vi "ReadCamera.vi"(7 "Color":u16(ring) items=["Blue", "Green", "Red", "Orange", "Yellow"], 8 "error in":errorcluster) -> (0 "error out":errorcluster, 2 "Camera Data":dbl[][](array[numeric]) format="%.2f")   [LabVIEW 2018]
uses:
  <vilib>/vision/NI_Vision_Development_Module.lvlib
panel:
  out "Image":T1(plugin-control)
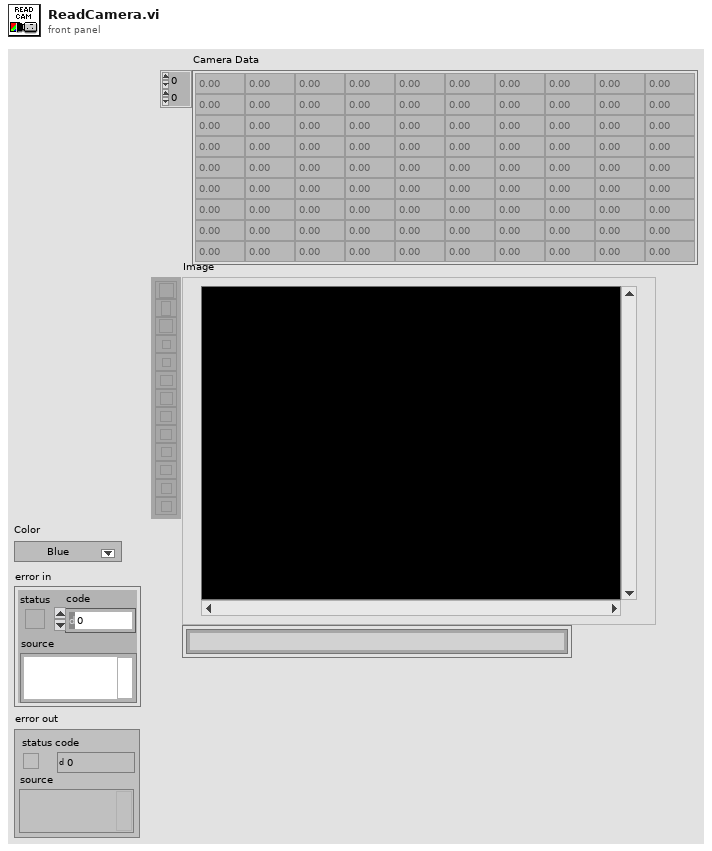
[diagram p1: front panel]
types:
  T1 = typedef "IMAQ Image.ctl" = refnum<image>
  T2 = typedef "Particle Parameters" = i32
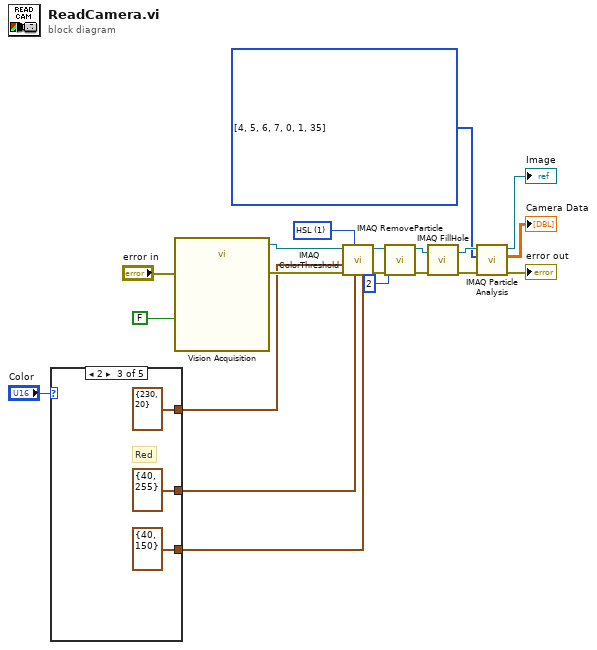
[diagram p0: block diagram]
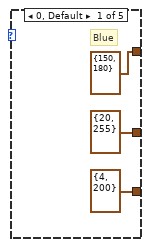
[diagram p2: hidden frame]
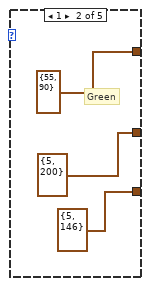
[diagram p3: hidden frame]
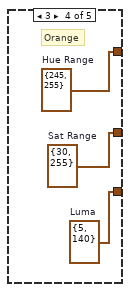
[diagram p4: hidden frame]
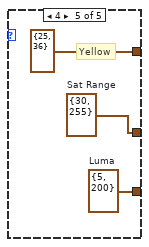
[diagram p5: hidden frame]
diagram:
  w7 = T2[] [4, 5, 6, 7, 0, 1, 35] items=["Center of Mass X", "Center of Mass Y", "First Pixel X", "First Pixel Y", "Bounding Rect Left", "Bounding Rect Top", "Bounding Rect Right", "Bounding Rect Bottom", "Max Feret Diameter Start X", "Max Feret Diameter Start Y", "Max Feret Diameter End X", "Max Feret Diameter End Y", "Max Horiz. Segment Length Left", "Max Horiz. Segment Length Right", "Max Horiz. Segment Length Row", "-", "Bounding Rect Width", "Bounding Rect Height", "Bounding Rect Diagonal", "Perimeter", "Convex Hull Perimeter", "Holes' Perimeter", "Max Feret Diameter", "Equivalent Ellipse Major Axis", "Equivalent Ellipse Minor Axis", "Equivalent Ellipse Minor Axis (Feret)", "Equivalent Rect Long Side", "Equivalent Rect Short Side", "Equivalent Rect Diagonal", "Equivalent Rect Short Side (Feret)", "Average Horiz. Segment Length", "Average Vert. Segment Length", "Hydraulic Radius", "Waddel Disk Diameter", "-", "Area", "Holes' Area", "Particle & Holes' Area", "Convex Hull Area", "Image Area", "-", "Number of Holes", "Number of Horiz. Segments", "Number of Vert. Segments", "-", "Orientation", "Max Feret Diameter Orientation", "-", "% Area/Image Area", "% Area/(Particle & Holes' Area)", "Ratio of Equivalent Ellipse Axes", "Ratio of Equivalent Rect Sides", "-", "Elongation Factor", "Compactness Factor", "Heywood Circularity Factor", "Type Factor", "-", "Sum X", "Sum Y", "Sum XX", "Sum XY", "Sum YY", "Sum XXX", "Sum XXY", "Sum XYY", "Sum YYY", "-", "Moment of Inertia XX", "Moment of Inertia XY", "Moment of Inertia YY", "Moment of Inertia XXX", "Moment of Inertia XXY", "Moment of Inertia XYY", "Moment of Inertia YYY", "Norm. Moment of Inertia XX", "Norm. Moment of Inertia XY", "Norm. Moment of Inertia YY", "Norm. Moment of Inertia XXX", "Norm. Moment of Inertia XXY", "Norm. Moment of Inertia XYY", "Norm. Moment of Inertia YYY", "Hu Moment 1", "Hu Moment 2", "Hu Moment 3", "Hu Moment 4", "Hu Moment 5", "Hu Moment 6", "Hu Moment 7"] ("Pixel Measurements")
  w17 = u16 1 items=["RGB", "HSL", "HSV", "HSI"] ("Color Mode")
  n1 = case shown="2" "Color" {
    tunnel: [cluster{"Lower value":i32, "Upper value":i32} {"Lower value"=150, "Upper value"=180} ("Hue Range") cluster{"Lower value":i32, "Upper value":i32} {"Lower value"=55, "Upper value"=90} ("Hue Range") cluster{"Lower value":i32, "Upper value":i32} {"Lower value"=230, "Upper value"=20} ("Hue Range") w32 cluster{"Lower value":i32, "Upper value":i32} {"Lower value"=25, "Upper value"=36} ("Hue Range")] -> w16
    tunnel: [cluster{"Lower value":i32, "Upper value":i32} {"Lower value"=20, "Upper value"=255} ("Sat Range") cluster{"Lower value":i32, "Upper value":i32} {"Lower value"=5, "Upper value"=200} ("Sat Range") cluster{"Lower value":i32, "Upper value":i32} {"Lower value"=40, "Upper value"=255} ("Sat Range") w31 w34] -> w15
    tunnel: [cluster{"Lower value":i32, "Upper value":i32} {"Lower value"=4, "Upper value"=200} ("Luma") cluster{"Lower value":i32, "Upper value":i32} {"Lower value"=5, "Upper value"=146} ("Luma") cluster{"Lower value":i32, "Upper value":i32} {"Lower value"=40, "Upper value"=150} ("Luma") w30 w33] -> w14
    frame 0, Default {
      # "Blue"
    }
    frame 1 {
      # "Green"
    }
    frame 2 {
      # "Red"
    }
    frame 3 {
      w30 = cluster{"Lower value":i32, "Upper value":i32} {"Lower value"=5, "Upper value"=140}  # Luma
      w31 = cluster{"Lower value":i32, "Upper value":i32} {"Lower value"=30, "Upper value"=255}  # Sat Range
      w32 = cluster{"Lower value":i32, "Upper value":i32} {"Lower value"=245, "Upper value"=255}  # Hue Range
      # "Orange"
    }
    frame 4 {
      w33 = cluster{"Lower value":i32, "Upper value":i32} {"Lower value"=5, "Upper value"=200}  # Luma
      w34 = cluster{"Lower value":i32, "Upper value":i32} {"Lower value"=30, "Upper value"=255}  # Sat Range
      # "Yellow"
    }
  }
  n2 = call "Vision Acquisition"("Stop (F)"=FALSE, "error in"="error in") -> ("Image Out"=w3:T1, "error out"=w18:errorcluster)  [unwired: 23 in, 1 out]
  n3 = call "IMAQ ColorThreshold"("Blue or Luma or Val or Inten Range"=w14, "Green or Sat Range"=w15, "Color Mode"=w17, "error in (no error)"=w18, "Red or Hue Range"=w16, "Image Src"=w3) -> ("error out"=w13:errorcluster, "Image Dst Out"=w12:T1)  [unwired: 4 in]
  n4 = call "IMAQ RemoveParticle"("error in (no error)"=w13, "Number of Erosion"=2, "Image Src"=w12) -> ("error out"=w11:errorcluster, "Image Dst Out"=w10:T1)  [unwired: 7 in]
  n5 = call "IMAQ FillHole"("error in (no error)"=w11, "Image Src"=w10) -> ("error out"=w9:errorcluster, "Image Dst Out"=w8:T1)  [unwired: 4 in]
  n6 = call "IMAQ Particle Analysis"("error in (no error)"=w9, "Pixel Measurements"=w7, "Image"=w8) -> ("error out"=→"error out":errorcluster, "Particle Measurements (Pixels)"=→"Camera Data":dbl[][], "Image Out (duplicate)"=→"Image":T1)  [unwired: 3 in, 3 out]
